vi "loop_data_labels.vi"() -> (0 "Loop Data Labels":string[](array[string])=["Timestamp", "Vap Mass Flow", "Liq Mass Flow", "DP", "Liq Tank P", "LiqTank T", "Sep P", "SepT", "Liq In P", "Liq In T", "Vap Tank P", "Vap Tank T", "Dev Section P", "Dev Section T", "Up TS P", "Up TS T", "Low TS P", "Low TS T", "Cond Top T", "Evap Top T", "Cond Bot T", "Evap Bot T", "Win 3-4 P", "Top Heat T", "Bot Heat T", ""])   [LabVIEW 2015]
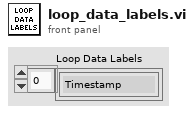
[diagram p1: front panel]
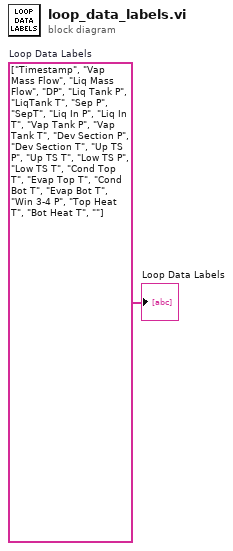
[diagram p0: block diagram]
diagram:
  w1 = string[] ["Timestamp", "Vap Mass Flow", "Liq Mass Flow", "DP", "Liq Tank P", "LiqTank T", "Sep P", "SepT", "Liq In P", "Liq In T", "Vap Tank P", "Vap Tank T", "Dev Section P", "Dev Section T", "Up TS P", "Up TS T", "Low TS P", "Low TS T", "Cond Top T", "Evap Top T", "Cond Bot T", "Evap Bot T", "Win 3-4 P", "Top Heat T", "Bot Heat T", ""]  # Loop Data Labels
  "Loop Data Labels" <- w1
